vi "set to range.vi"(4 "kąt [rad]":dbl) -> (1 "kąt [rad] zredukowany":dbl)   [LabVIEW 2015]
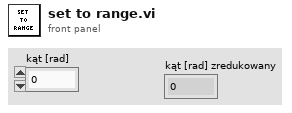
[diagram p1: front panel]
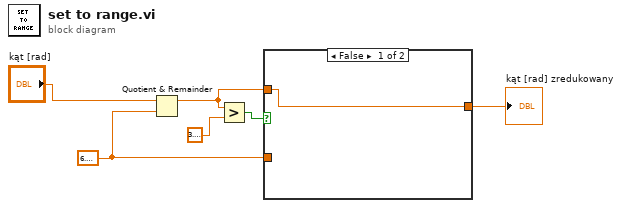
[diagram p0: block diagram]
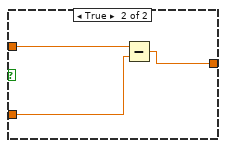
[diagram p2: hidden frame]
diagram:
  w2 = 6.283185307179586
  n1 = Quotient & Remainder(x="kąt [rad]", y=w2) -> (x-y*floor(x/y)=w3:dbl)  [unwired: 1 out]
  n2 = Greater?(x=w3, y=3.141592653589793) -> (0:w5:bool)
  n3 = case shown="False" w5 {
    tunnel: w3 -> [w7 w10]
    tunnel: w2 -> [_ w9]
    tunnel: [w7 w8] -> w1
    frame False {
    }
    frame True {
      n4 = Subtract(x=w10, y=w9) -> (x-y=w8:dbl)
    }
  }
  "kąt [rad] zredukowany" <- w1
